vi "main_load_environment_check.vi"(10 "New working Dir":path) -> (0 "Num_Hydro":string, 1 "Structure":string, 2 "Valid?":bool, 3 "Endtime":string, 4 "FlowVal":string)   [LabVIEW 2019]
uses:
  <vilib>/regexp/Match Regular Expression.xnode
panel:
  out "Starttime":string
  out "Finished?":string
  # "*******************************************************************\nBiogas Plant Control\n\nAuthor: Paul Zügel\nGCSC-Frankfurt am Main 2020\n\n*******************************************************************"
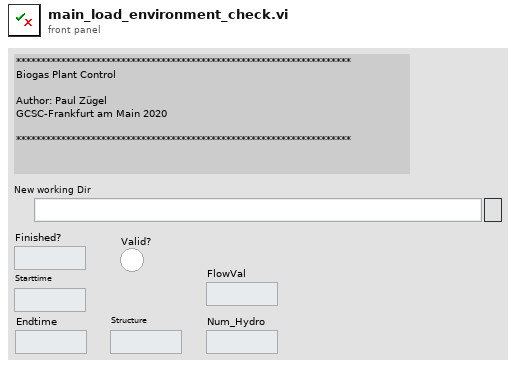
[diagram p1: front panel]
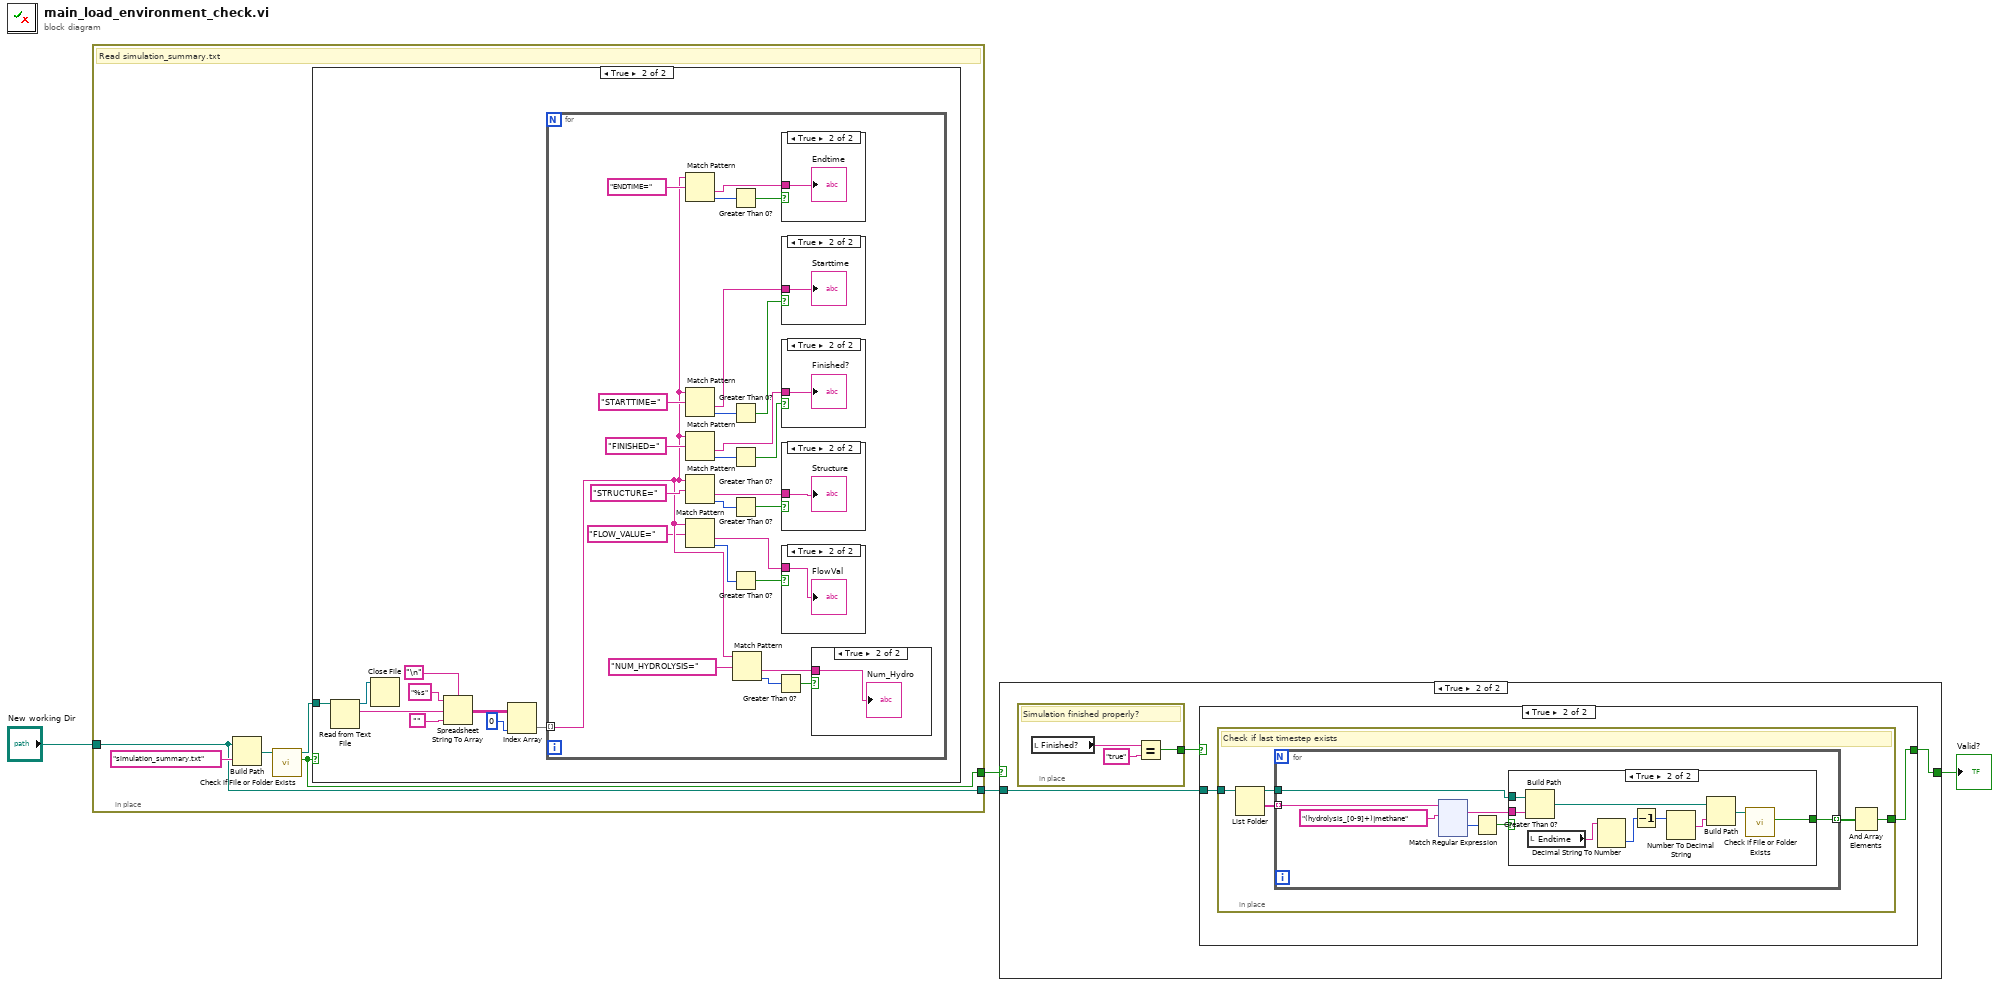
[diagram p0: block diagram]
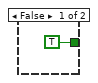
[diagram p4: hidden frame]
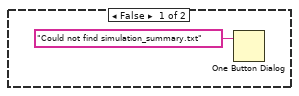
[diagram p5: hidden frame]
diagram:
  n1 = in-place {
    in-place-border: [w7] -> w1
    in-place-border: "New working Dir" -> [w5]
    in-place-border: [w5] -> w2
    # "Read simulation_summary.txt"
    n2 = Build Path(base path=w5, name or relative path="simulation_summary.txt") -> (appended path=w6:path)
    n3 = call <vilib>:"Check if File or Folder Exists.vi"("path"=w6) -> ("file or folder exists?"=w7:bool, "dup path"=w8:path)  [unwired: 8 in, 1 out]
    n4 = case shown="True" w7 {
      tunnel: w8 -> [_ w19]
      frame False {
        n5 = One Button Dialog(message="Could not find simulation_summary.txt") -> ()  [unwired: 1 in, 1 out]
      }
      frame True {
        n6 = Read from Text File(file (use dialog)=w19) -> (refnum out=w11:refnum<file>, text=w18:string)  [unwired: 3 in, 2 out]
        n7 = Close File(refnum=w11) -> ()  [unwired: 1 in, 2 out]
        n8 = Spreadsheet String To Array(delimiter (Tab)="\n", format string="%s", spreadsheet string=w18, array type (2D Dbl)="") -> (array=w12:string[][])
        n9 = Index Array(array=w12, index (col)=0 ("disabled index (col)")) -> (element=w13:string[])  [unwired: 1 in]
        n10 = for {
          tunnel: w13 -> [w21] mode=indexing
          n11 = Match Pattern(string=w21, regular expression="ENDTIME=") -> (after substring=w39:string, offset past match=w34:i32)  [unwired: 1 in, 2 out]
          n12 = Match Pattern(string=w21, regular expression="STARTTIME=") -> (after substring=w41:string, offset past match=w36:i32)  [unwired: 1 in, 2 out]
          n13 = Match Pattern(string=w21, regular expression="FINISHED=") -> (after substring=w43:string, offset past match=w38:i32)  [unwired: 1 in, 2 out]
          n14 = Match Pattern(string=w21, regular expression="STRUCTURE=") -> (after substring=w31:string, offset past match=w30:i32)  [unwired: 1 in, 2 out]
          n15 = Match Pattern(string=w21, regular expression="FLOW_VALUE=") -> (after substring=w23:string, offset past match=w24:i32)  [unwired: 1 in, 2 out]
          n16 = Greater Than 0?(x=w34) -> (x > 0?=w33:bool)
          n17 = Greater Than 0?(x=w36) -> (x > 0?=w35:bool)
          n18 = Greater Than 0?(x=w38) -> (x > 0?=w37:bool)
          n19 = Greater Than 0?(x=w30) -> (x > 0?=w29:bool)
          n20 = Greater Than 0?(x=w24) -> (x > 0?=w22:bool)
          n21 = Match Pattern(string=w21, regular expression="NUM_HYDROLYSIS=") -> (after substring=w27:string, offset past match=w26:i32)  [unwired: 1 in, 2 out]
          n22 = Greater Than 0?(x=w26) -> (x > 0?=w25:bool)
          n23 = case shown="True" w33 {
            tunnel: w39 -> [_ w50]
            frame False {
            }
            frame True {
              "Endtime" <- w50
            }
          }
          n24 = case shown="True" w35 {
            tunnel: w41 -> [_ w49]
            frame False {
            }
            frame True {
              "Starttime" <- w49
            }
          }
          n25 = case shown="True" w37 {
            tunnel: w43 -> [_ w48]
            frame False {
            }
            frame True {
              "Finished?" <- w48
            }
          }
          n26 = case shown="True" w29 {
            tunnel: w31 -> [_ w47]
            frame False {
            }
            frame True {
              "Structure" <- w47
            }
          }
          n27 = case shown="True" w22 {
            tunnel: w23 -> [_ w45]
            frame False {
            }
            frame True {
              "FlowVal" <- w45
            }
          }
          n28 = case shown="True" w25 {
            tunnel: w27 -> [_ w46]
            frame False {
            }
            frame True {
              "Num_Hydro" <- w46
            }
          }
        }
      }
    }
  }
  n29 = case shown="True" w1 {
    selector: w1 -> [w51 _]
    tunnel: [w51 w54] -> w4
    tunnel: w2 -> [_ w53]
    frame False {
    }
    frame True {
      n30 = in-place {
        in-place-border: [w194] -> w52
        # "Simulation finished properly?"
        n31 = local read "Finished?"() -> (w196:string)
        n32 = Equal?(x=w196, y="true") -> (x = y?=w194:bool)
      }
      n33 = case shown="True" w52 {
        selector: w52 -> [w55 _]
        tunnel: [w55 w57] -> w54
        tunnel: w53 -> [_ w56]
        frame False {
        }
        frame True {
          n34 = in-place {
            in-place-border: [w62] -> w57
            in-place-border: w56 -> [w61]
            # "Check if last timestep exists"
            n35 = List Folder(path=w61) -> (path out=w59:path, folder names=w60:string[])  [unwired: 3 in, 2 out]
            n36 = for {
              tunnel: w60 -> [w68] mode=indexing
              tunnel: w59 -> [w65]
              tunnel: [w63] -> w58 mode=indexing
              n37 = xnode "Match Regular Expression"("input string"=w68, "regular expression"="(hydrolysis_[0-9]+)|methane") -> ("whole match"=w64:string, "offset past match"=w67:i32)  [unwired: 4 in, 3 out]
              n38 = Greater Than 0?(x=w67) -> (x > 0?=w66:bool)
              n39 = case shown="True" w66 {
                tunnel: w65 -> [_ w79]
                tunnel: w64 -> [_ w78]
                tunnel: [TRUE w75] -> w63
                frame False {
                }
                frame True {
                  n40 = Build Path(base path=w79, name or relative path=w78) -> (appended path=w77:path)
                  n41 = local read "Endtime"() -> (w74:string)
                  n42 = Decimal String To Number(string=w74) -> (number=w73:i32)  [unwired: 2 in, 1 out]
                  n43 = Decrement(x=w73) -> (x-1=w72:i32)
                  n44 = Number To Decimal String(number=w72) -> (decimal integer string=w71:string)  [unwired: 1 in]
                  n45 = Build Path(base path=w77, name or relative path=w71) -> (appended path=w76:path)
                  n46 = call <vilib>:"Check if File or Folder Exists.vi"("path"=w76) -> ("file or folder exists?"=w75:bool)  [unwired: 8 in, 2 out]
                }
              }
            }
            n47 = And Array Elements(Boolean array=w58) -> (logical AND=w62:bool)
          }
        }
      }
    }
  }
  "Valid?" <- w4
